vi "加载OBD.vi"(8 "error in (no error)":errorcluster caption="错误输入（无错误）") -> (0 "error out":errorcluster caption="错误输出")   [LabVIEW 2014]
doc: "该模板用于创建子VI。"
uses:
  glb/glb_data.vi
  glb/glb_static.vi
  <vilib>/Utility/config.llb/NI_LVConfig.lvlib
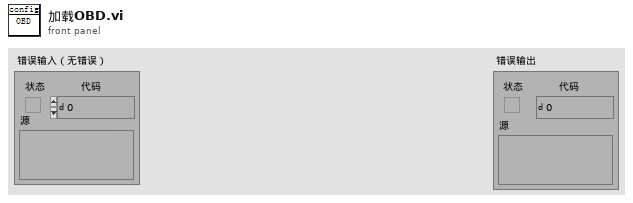
[diagram p1: front panel]
types:
  T1 = typedef "NI_LVConfig.lvlib/Config Data RefNum.ctl" = refnum<k1>
  T2 = cluster{"名称":string, "简称":string, "单位":string, "附加":string[], "类型":enum16{"测试模块", "FPGA", "cRIO", "其他设备", "总体展示"}}
  T3 = cluster{"串口资源名称":string, "波特率":u32, "数据比特":u32, "奇偶":u32, "停止位":u32, "流控制":u32, "超时":u32}
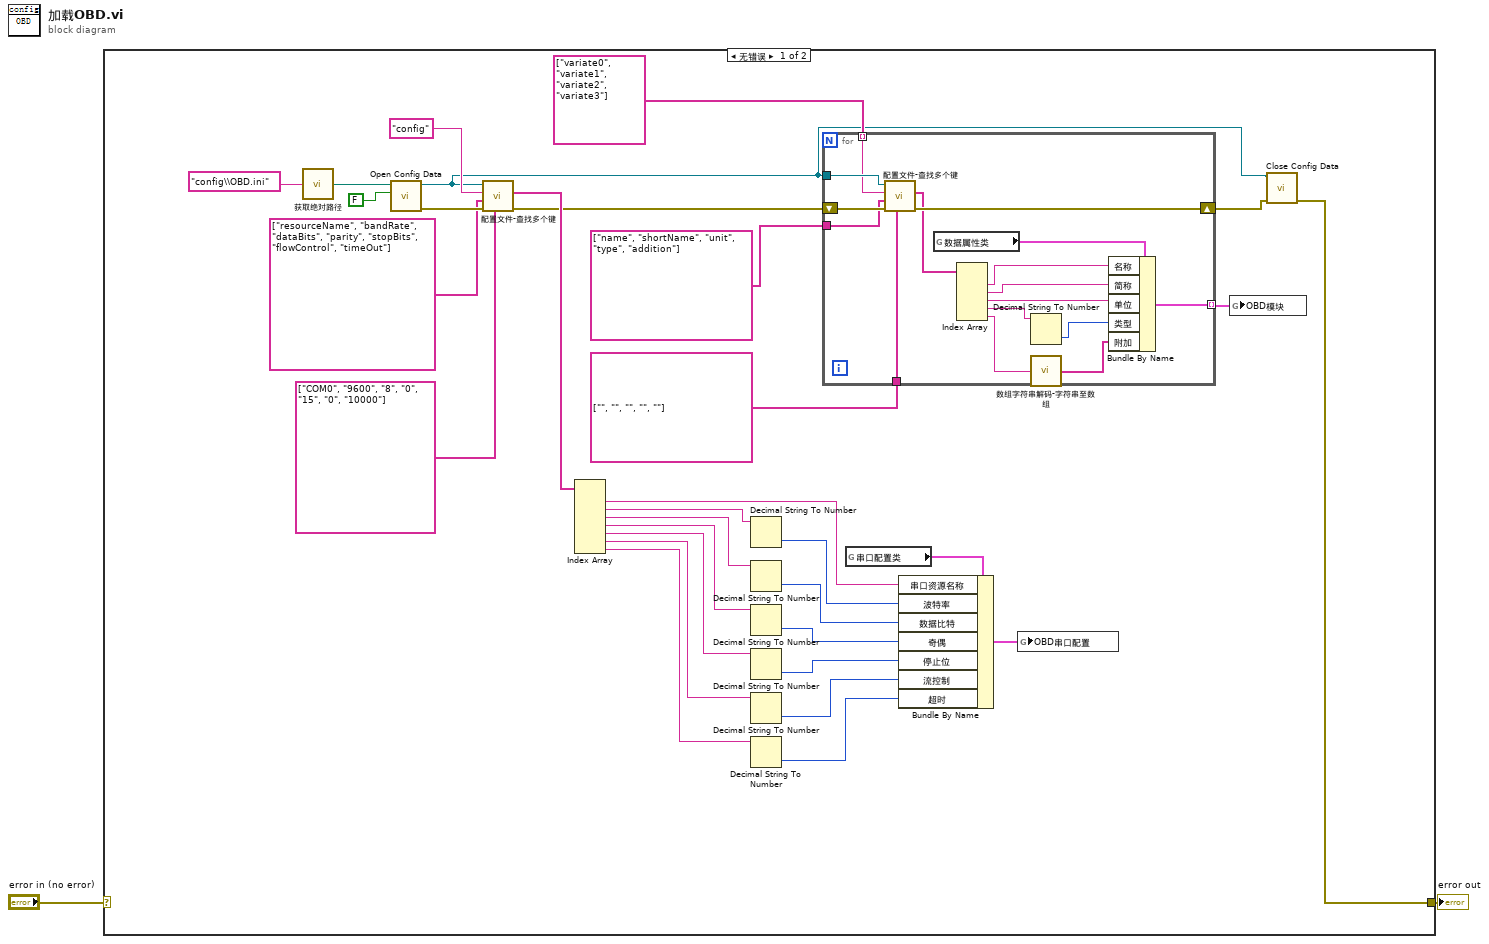
[diagram p0: block diagram]
diagram:
  n1 = case shown="无错误" "error in (no error)" {
    selector: "error in (no error)" -> [_ w50]
    tunnel: [w4 w50] -> w1
    frame No Error {
      n2 = call "获取绝对路径.vi"("relativePath"="config\\OBD.ini") -> ("absolutePath"=w32:path)
      n3 = call <vilib>:"Open Config Data.vi"("create file if necessary (T)"=FALSE, "configuration file path"=w32) -> ("error out"=w30:errorcluster, "refnum"=w5:T1)  [unwired: 7 in, 1 out]
      n4 = call "配置文件-查找多个键.vi"("默认值"=string[] ["COM0", "9600", "8", "0", "15", "0", "10000"], "错误输入（无错误）"=w30, "键名"=string[] ["resourceName", "bandRate", "dataBits", "parity", "stopBits", "flowControl", "timeOut"], "章名"="config", "引用句柄输入"=w5) -> ("错误输出"=w10:errorcluster, "查询结果"=w25:string[])  [unwired: 4 in, 1 out]
      n5 = Index Array(array=w25) -> (element #1=w24:string, element #2=w23:string, element #3=w21:string, element #4=w19:string, element #5=w17:string, element #6=w15:string, element #7=w13:string)  [unwired: 7 in]
      n6 = Decimal String To Number(string=w23) -> (number=w22:i32)  [unwired: 2 in, 1 out]
      n7 = Decimal String To Number(string=w21) -> (number=w20:i32)  [unwired: 2 in, 1 out]
      n8 = Decimal String To Number(string=w19) -> (number=w18:i32)  [unwired: 2 in, 1 out]
      n9 = Decimal String To Number(string=w17) -> (number=w16:i32)  [unwired: 2 in, 1 out]
      n10 = Decimal String To Number(string=w15) -> (number=w14:i32)  [unwired: 2 in, 1 out]
      n11 = Decimal String To Number(string=w13) -> (number=w12:i32)  [unwired: 2 in, 1 out]
      n12 = for {
        tunnel: w5 -> [w48]
        tunnel: string[] ["variate0", "variate1", "variate2", "variate3"] -> [w47] mode=indexing
        tunnel: string[] ["name", "shortName", "unit", "type", "addition"] -> [w46]
        tunnel: string[] ["", "", "", "", ""] -> [w45]
        shift-right: [w44] -> w6
        shift-left: w10 -> [w49]
        tunnel: [w34] -> w3 mode=indexing
        n13 = call "配置文件-查找多个键.vi"("默认值"=w45, "错误输入（无错误）"=w49, "键名"=w46, "章名"=w47, "引用句柄输入"=w48) -> ("错误输出"=w44:errorcluster, "查询结果"=w35:string[])  [unwired: 4 in, 1 out]
        n14 = global read "类信息.vi" "数据属性类"() -> (w43:T2)
        n15 = Index Array(array=w35) -> (element #1=w42:string, element #2=w41:string, element #3=w40:string, element #4=w39:string, element #5=w37:string)  [unwired: 5 in]
        n16 = Decimal String To Number(string=w39) -> (number=w38:i32)  [unwired: 2 in, 1 out]
        n17 = call "数组字符串解码-字符串至数组.vi"("字符串"=w37) -> ("数组"=w36:string[])  [unwired: 1 in]
        n18 = Bundle By Name(cluster=w43, "名称"=w42, "简称"=w41, "单位"=w40, "类型"=w38, "附加"=w36) -> (w34:T2)
      }
      n19 = global read "类信息.vi" "串口配置类"() -> (w26:T3)
      n20 = Bundle By Name(cluster=w26, "串口资源名称"=w24, "波特率"=w22, "数据比特"=w20, "奇偶"=w18, "停止位"=w16, "流控制"=w14, "超时"=w12) -> (w11:T3)
      n21 = global write "glb_static.vi" "OBD串口配置"(w11) -> ()
      n22 = global write "glb_data.vi" "OBD模块"(w3) -> ()
      n23 = call <vilib>:"Close Config Data.vi"("error in (no error)"=w6, "refnum"=w5) -> ("error out"=w4:errorcluster)  [unwired: 8 in, 1 out]
    }
    frame Error {
    }
  }
  "error out" <- w1
